vi "array_generator.vi"(0 "Index":i32, 1 "Array":u8[](array[numeric])=[0, 0, 0, 0, 0, 0, 0, 0]) -> (2 "Boolean array":bool[](array[boolean]))   [LabVIEW 2019]
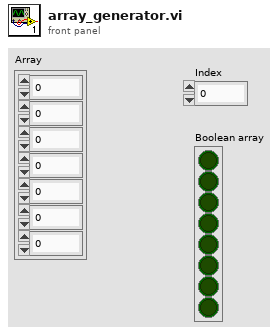
[diagram p1: front panel]
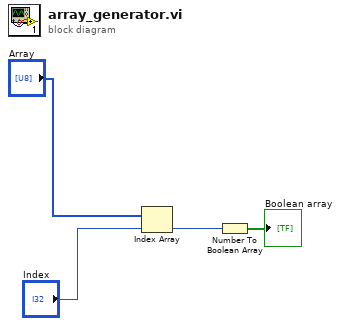
[diagram p0: block diagram]
diagram:
  n1 = Index Array(array="Array", index="Index") -> (element=w2:u8)
  n2 = Number To Boolean Array(number=w2) -> (Boolean array=→"Boolean array":bool[])
